vi "Handle Error.vi"(8 "error in (no error)":errorcluster, 11 "VisionUI in":refnum<class "VisionUI.lvclass">) -> (0 "error out":errorcluster, 2 "stop actor?":bool=TRUE, 3 "VisionUI out":refnum<class "VisionUI.lvclass">)   [LabVIEW 2019, in "VisionUI.lvlib" / "VisionUI.lvclass"]
doc: "(<B>Filename</B>: Actor Framework.lvlib:Actor.lvclass:Handle Error.vi)\n\nDefines how the actor handles an error that occurred while processing a message. By default, this method does nothing except stop the actor."
uses:
  VisionUI.lvclass
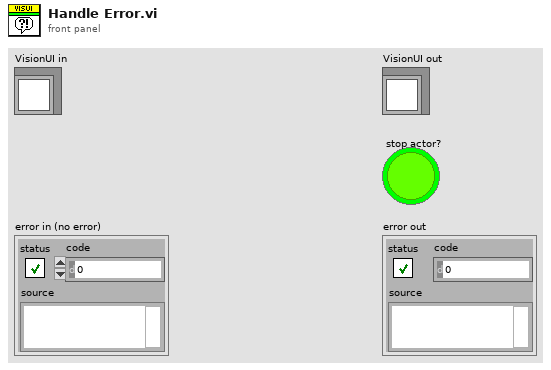
[diagram p1: front panel]
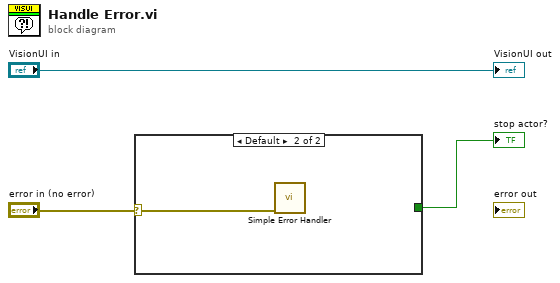
[diagram p0: block diagram]
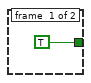
[diagram p2: hidden frame]
diagram:
  n1 = case shown="Default" "error in (no error)" {
    selector: "error in (no error)" -> [_ w5]
    tunnel: [TRUE _] -> w1
    frame #0 {
    }
    frame #1 {
      n2 = call <vilib>:"Simple Error Handler.vi"("error in (no error)"=w5) -> ()  [unwired: 4 in, 5 out]
    }
  }
  "stop actor?" <- w1
  "VisionUI out" <- "VisionUI in"
